vi "Create gplugindata file.vi"(8 "error in":errorcluster, 9 "gplugindata in":string, 10 "Library":string, 11 "Destination Path":path) -> (0 "error out":errorcluster)   [LabVIEW 2021, in "CIF Build Actions.lvlib"]
uses:
  CIF Build Actions.lvlib
  CIFCore/Common/Typedef/Errors.ctl
  <vilib>/CIF Foundation/CIF Utilities/Errors/Append Error Location.vi
  CIFCore/Common/CIFCoreCommon.lvlib
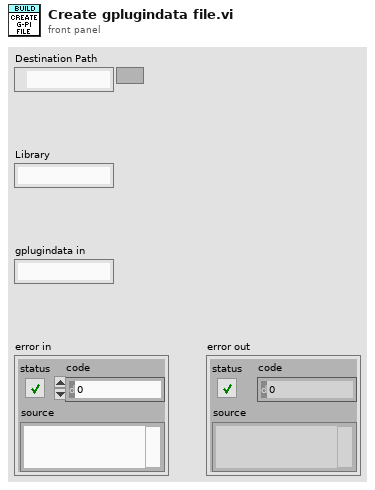
[diagram p1: front panel]
types:
  T1 = typedef "CIFCoreCommon.lvlib/Errors.ctl" = enum16{"Invalid Clock ID", "Long Sleep", "gRPC Server Not Found", "Config Parse", "Timestamp Wrap", "Delayed Execution", "Duplicate Channel", "Missing Channel", "Incorrect Type", "Flatten Error", "Unflatten Data", "Unique Name", "Plugin Not Found", "Plugin Type Not Found", "Plugin Version Not Found", "Manager Not Found", "Numerical Issue", "Time Jump", "Clock ID Match", "Channel Length", "Plugin Connection", "gRPC Server Connection", "PPL Name Match", "Build", "Config Log Parse", "Plugin Load", "UI Subpanel Load", "Python Name", "Invalid Name"}
  T2 = enum16{"open", "replace", "create", "open or create", "replace or create", "replace or create with confirmation"}
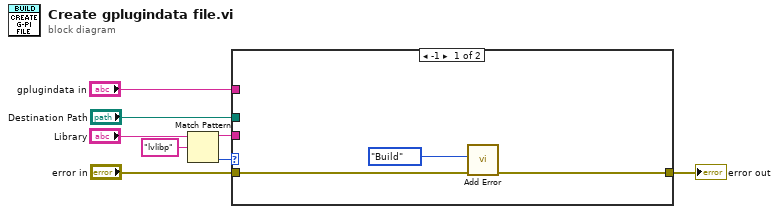
[diagram p0: block diagram]
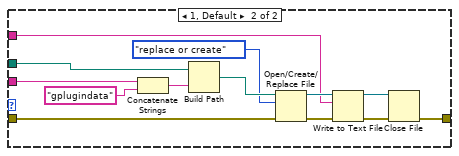
[diagram p2: hidden frame]
diagram:
  n1 = Match Pattern(string="Library", regular expression="lvlibp") -> (before substring=w6:string, offset past match=w4:i32)  [unwired: 1 in, 2 out]
  n2 = case shown="-1" w4 {
    tunnel: w6 -> [_ w24]
    tunnel: "Destination Path" -> [_ w21]
    tunnel: "error in" -> [w11 w18]
    tunnel: "gplugindata in" -> [_ w15]
    tunnel: [w10 w12] -> w1
    frame -1 {
      n3 = call "Add Error.vi"("error in (no error)"=w11, "Error"=Errors."Build") -> ("error out"=w10:errorcluster)  [unwired: 9 in]
    }
    frame 1, Default {
      n4 = Concatenate Strings(w24, "gplugindata" ("string")) -> (w22:string)
      n5 = Build Path(base path=w21, name or relative path=w22) -> (appended path=w20:path)
      n6 = Open/Create/Replace File(file path (use dialog)=w20, error in=w18, operation (0:open)=T2."replace or create") -> (refnum out=w17:refnum<file>, error out=w16:errorcluster)  [unwired: 3 in, 1 out]
      n7 = Write to Text File(file (use dialog)=w17, text=w15, error in=w16) -> (refnum out=w14:refnum<file>, error out=w13:errorcluster)  [unwired: 1 in, 1 out]
      n8 = Close File(refnum=w14, error in=w13) -> (error out=w12:errorcluster)  [unwired: 1 out]
    }
  }
  "error out" <- w1
